vi "Configure Basic Multitone.vi"(0 "VISA resource name":refnum<visa-resource-name>, 1 "Invert EQ (T: Enable)":bool=TRUE, 2 "Enable Analyze Noise (F: Disabled)":bool, 5 "Analyzer (0: A0)":i32(ring) items=["A0", "A1"], 7 "Processing (0: mpSync)":i32(ring) items=["mpSync", "mpWindow"], 9 "FFT Window (0: fftBlackmanHarris)":i32(ring) items=["fftBlackmanHarris", "fftHann", "fftHamming", "fftEquiripple", "fftFlattop", "fftGaussian", "fftKaiser", "fftUniform", "fftRifeVincent4", "fftRifeVincent5", "fftRifeVincent10", "fftBlackmanHarris7"], 11 "error in (no error)":errorcluster, 12 "Relative Mode (0: mtAbsolute)":i32(ring) items=["mtAbsolute", "mtRelGen", "mtRelGenOther", "mtRelTone", "mtRelToneOther", "mtRelTotal"]) -> (4 "VISA resource name out":refnum<visa-resource-name>, 15 "error out":errorcluster)   [LabVIEW 2014, in "Stanford Research SR1.lvlib"]
doc: "Configures the basic attributes for the Multitone Analyzer."
uses:
  Stanford Research SR1.lvlib
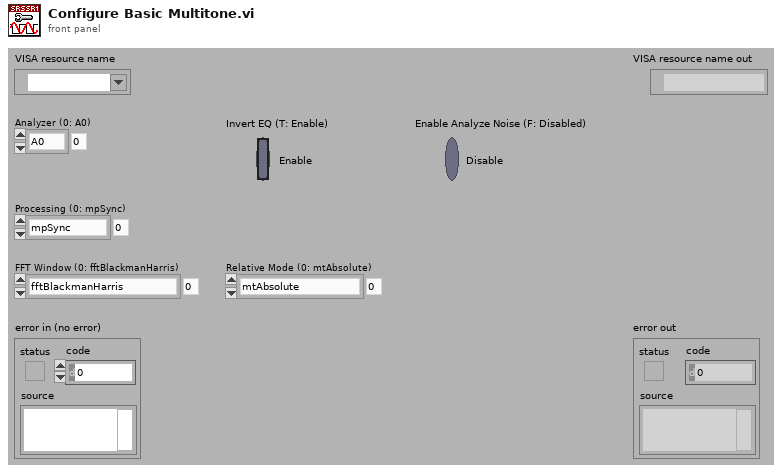
[diagram p1: front panel]
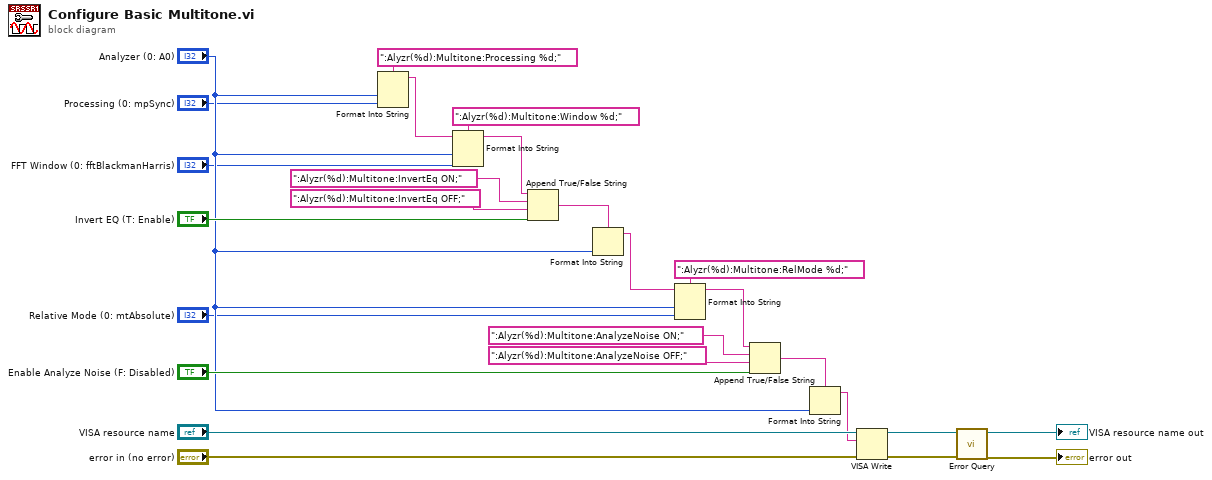
[diagram p0: block diagram]
diagram:
  n1 = Format Into String(format string=":Alyzr(%d):Multitone:Processing %d;", "Analyzer (0: A0)", "Processing (0: mpSync)") -> (resulting string=w25:string)  [unwired: 2 in, 1 out]
  n2 = Format Into String(format string=":Alyzr(%d):Multitone:Window %d;", initial string=w25, "Analyzer (0: A0)", "FFT Window (0: fftBlackmanHarris)") -> (resulting string=w23:string)  [unwired: 1 in, 1 out]
  n3 = Append True/False String(1:"Invert EQ (T: Enable)", 2:":Alyzr(%d):Multitone:InvertEq OFF;", 3:":Alyzr(%d):Multitone:InvertEq ON;", 4:w23) -> (0:w8:string)
  n4 = Format Into String(format string=w8, "Analyzer (0: A0)") -> (resulting string=w7:string)  [unwired: 2 in, 1 out]
  n5 = Format Into String(format string=":Alyzr(%d):Multitone:RelMode %d;", initial string=w7, "Analyzer (0: A0)", "Relative Mode (0: mtAbsolute)") -> (resulting string=w18:string)  [unwired: 1 in, 1 out]
  n6 = Append True/False String(1:"Enable Analyze Noise (F: Disabled)", 2:":Alyzr(%d):Multitone:AnalyzeNoise OFF;", 3:":Alyzr(%d):Multitone:AnalyzeNoise ON;", 4:w18) -> (0:w6:string)
  n7 = Format Into String(format string=w6, "Analyzer (0: A0)") -> (resulting string=w5:string)  [unwired: 2 in, 1 out]
  n8 = VISA Write(VISA resource name="VISA resource name", write buffer=w5, error in (no error)="error in (no error)") -> (VISA resource name out=w12:refnum<visa-resource-name>, error out=w11:errorcluster)  [unwired: 1 out]
  n9 = call "Error Query.vi"("error in (no error)"=w11, "VISA resource name"=w12) -> ("error out"=→"error out":errorcluster, "VISA resource name out"=→"VISA resource name out":refnum<visa-resource-name>)  [unwired: 6 in, 2 out]
